vi "Change Delimiters.vi"(8 "Error In":errorcluster, 11 "Parser In":refnum<class "Parser.lvclass">) -> (0 "Error Out":errorcluster, 3 "Parser Out":refnum<class "Parser.lvclass">)   [LabVIEW 2018, in "Mustache.lvlib" / "Parser.lvclass"]
uses:
  Parser.lvclass
  Parser.lvclass/Parser.ctl
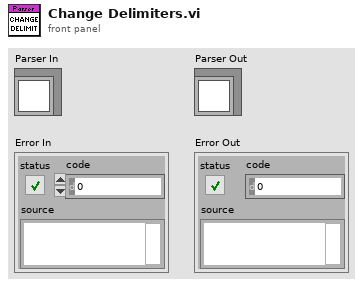
[diagram p1: front panel]
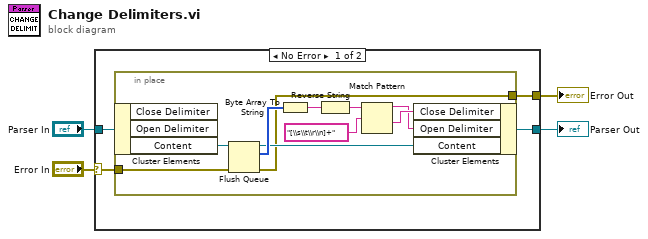
[diagram p0: block diagram]
diagram:
  n1 = case shown="No Error" "Error In" {
    selector: "Error In" -> [w5 w19]
    tunnel: [w8 w19] -> w4
    tunnel: [w7 w20] -> w3
    tunnel: "Parser In" -> [w6 w20]
    frame No Error {
      n2 = in-place {
        in-place-border: [w14] -> w8
        in-place-border: w5 -> [w9]
        n3 = in-place-cluster #1(w6) -> ("Content"=w18:refnum<queue>)  [unwired: 2 out]
        n4 = Flush Queue(queue=w18, error in (no error)=w9) -> (queue out=w15:refnum<queue>, remaining elements=w17:u8[], error out=w14:errorcluster)
        n5 = Byte Array To String(unsigned byte array=w17) -> (string=w16:string)
        n6 = Reverse String(1:w16) -> (0:w13:string)
        n7 = Match Pattern(string=w13, regular expression="[\\s\\t\\r\\n]+") -> (before substring=w10:string, after substring=w11:string)  [unwired: 1 in, 2 out]
        n8 = in-place-cluster #1("Close Delimiter"=w11, "Open Delimiter"=w10, "Content"=w15) -> (w7:refnum<class "Parser.lvclass">)
      }
    }
    frame Error {
    }
  }
  "Error Out" <- w4
  "Parser Out" <- w3
